vi "main.vi"() -> ()   [LabVIEW 2013]
uses:
  measure/meas session.ctl
  measure/Meas Sweep Config.ctl
  measure/Meas Freq Info.ctl
  measure/meas_swp_mode.ctl
  measure/meas_sweep_flist_mode.ctl
  bridge/Bridge Session.ctl
  bridge/Bridge Type.ctl
  drivers/TWM client/TWM Session.ctl
  drivers/TWM client/TWM parameters.ctl
  drivers/TWM client/Meas Proc QWTB Uncertainty Mode.ctl
  source/Source Session.ctl
  source/Source Type.ctl
  drivers/AFG3101C/AFG3101C Session.ctl
  drivers/cDAQ DDS/cDAQ DDS Session.ctl
  drivers/cDAQ DDS/cDAQ DDS Setup.ctl
  drivers/Fluke 5XXX/top_lev/F5xxx_session.ctl
  drivers/Fluke 5XXX/top_lev/F5xxx_output_mode.ctl
  measure/Meas Results.ctl
  bridge/Bridge Frequency Readings Data.ctl
  drivers/TWM client/Meas Proc QWTB Spectrum Data.ctl
  measure/Meas Result GUI References.ctl
  measure/Meas Result Freq Format.ctl
  measure/Meas Results Sweep Data Uncertainty Mode.ctl
  measure/Meas Result 4TP Impedance Mode.ctl
  measure/Meas Result Major Format.ctl
  measure/Meas Result Deviation Format.ctl
  varilib/SGUI Assign References Mode.ctl
  varilib/SGUI Assign Multiple Strings With Tags By Label.vi
  varilib/varilib.lvlib
panel:
  in  "mode 4TP":T1 caption="4TP display mode"
  in  "unc mode":T2 caption="Uncertainty display mode"
  in  "res frq fmt":T3
  in  "mnr dev fmt":T4 caption="Enum"
  in  "mjr dev fmt":T4 caption="Enum"
  in  "mnr fmt":T5=enum."%_5p"
  in  "mjr fmt":T5=enum."%_5p"
  out "tab swp":string[][](table) caption="Sweep data"
  out "gui refs":T6
  in  "results":T7
  out "meas ref":refnum<vi>
  in  "grp tabs":enum32{"Z", "Z(f)", "FFT", "Info"}(tab)
  out "grp Z mnr":dbl[](graph) caption="minor"
  out "grp Z mjr":dbl[](graph) caption="major"
  in  "swp mnr log":bool caption="Log"
  out "grp swp Z mnr":cluster{dbl[], dbl[]}[](graph) caption="minor"
  out "grp swp Z mjr":cluster{dbl[], dbl[]}[](graph) caption="major"
  in  "swp mjr log":bool caption="Log"
  out "grp ref":string
  out "grp spec 1":cluster{dbl[], dbl[]}(graph) caption="Amplitude spectrum for chn. 1"
  out "grp spec 0":cluster{dbl[], dbl[]}(graph) caption="Amplitude spectrum for chn. 0"
  in  "cb spec log":bool=TRUE caption="Log frequency"
  out "idn src":string caption="Source identifier"
  out "idn brg":string caption="Bridge/digitizers identifier"
  out "open cor":string caption="Open correction file"
  out "short cor":string caption="Short correction file"
  in  "swp com":string caption="Measurement comment"
  out "cab cor":string caption="Cable correction file"
  out "mpx cor":string caption="Multiplexer correction file"
  in  "fgen volts":string[][](table)=[["", "", ""]] caption="F-gen voltages"
  in  "meas":T10={"swp cfg"={"N"=0, "R"=0, "f list"=[], "smpl delay"=0.0, "set delay"=0.0, "set delay np"=0.0, "meas root"=path "", "meas name"="", "meas a-index"=FALSE, "rnd sweep"=FALSE, "mode"=enum."Frequency", "swp mode"=enum."Linear", "avg"=0, "subrec"=0}, "bridge"={"type"=enum."TWM client", "TWM"={"pipe name"="", "parameters"=[], "handle"=0, "fixed aper [s]"=0.0, "f-list [Hz]"=[], "discrete f-list"=FALSE, "unc mode"=enum."None", "unc mcc"=0, "unc first"=FALSE}, "last f"=0.0}, "src"={"type"=enum."Tektronix AFG3101C", "afg"={"VISA"="", "const"=0.0, "gen DC"=FALSE}, "cDAQ dds"={"device"="", "channels"=[], "mclk source"="", "mclk [Hz]"=0.0, "use ext mclk"=FALSE, "fs [Hz]"=0.0, "block [s]"=0.0, "buf [s]"=0.0, "task"="", "cmd queue"=refnum, "proc ref"=refnum, "smpl clock out"="/cDAQ3/PFI0", "export smpl clock"=FALSE}, "gain [V/A]"=1.0, "F5xxx session"={"VISA"="", "mode"=enum."AC voltage", "Earth on"=FALSE, "Ext ref lock"=FALSE}}, "results"=refnum} {"src"."cDAQ dds"."channels" min=0 step=1; "bridge"."TWM"."f-list [Hz]" format="%#_6p"; "swp cfg"."f list"."bias" format="%#_3p"; "swp cfg"."f list"."level" format="%#_3p"; "swp cfg"."f list"."fs [Hz]" format="%#_5p"; "swp cfg"."f list"."time [s]" format="%#_3p"; "swp cfg"."f list"."f/fs" format="%#_3p"; "swp cfg"."f list"."periods" format="%#_3f"; "swp cfg"."f list"."f [Hz]" format="%#_5p"}
  out "error":errorcluster
  in  "btn exit":bool
  in  "btn set&start":bool
  in  "btn cfg src":bool
  in  "btn cfg adc":bool
  in  "btn stop":bool
  out "stat3":string
  out "stat2":string
  out "stat1":string
  in  "btn about":bool
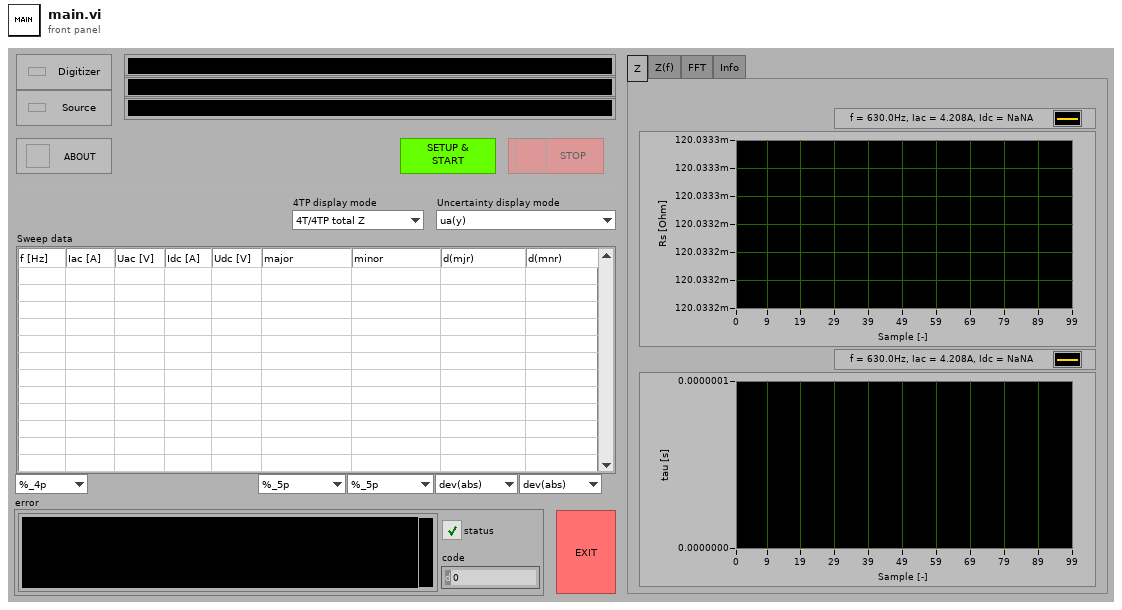
[diagram p1: front panel]
types:
  T1 = typedef "Meas Result 4TP Impedance Mode.ctl" = enum16{"4T/4TP total Z", "4TP-shield Z"}
  T2 = typedef "Meas Results Sweep Data Uncertainty Mode.ctl" = enum16{"ua(y)", "ua(y) (p=95%)", "uc(y) (p=95%)"}
  T3 = typedef "Meas Result Freq Format.ctl" = enum16{"%_4p", "%_4f"}
  T4 = typedef "Meas Result Deviation Format.ctl" = enum16{"dev(abs)", "dev(%)", "dev(ppm)", "u(abs)", "u(%)", "u(ppm)"}
  T5 = typedef "Meas Result Major Format.ctl" = enum16{"%_3p", "%_4p", "%_5p", "%_6p", "%_7p", "%_8p", "%_5f", "%_6f", "%_7f", "%_8f"}
  T6 = typedef "Meas Result GUI References.ctl" = cluster{"grp Z mjr":refnum<vi>, "grp Z mnr":refnum<vi>, "grp swp Z mjr":refnum<vi>, "grp swp Z mnr":refnum<vi>, "swp mjr log":refnum<vi>, "swp mnr log":refnum<vi>, "grp ref":refnum<vi>, "tab swp":refnum<vi>, "mjr fmt":refnum<vi>, "mnr fmt":refnum<vi>, "mjr dev fmt":refnum<vi>, "mnr dev fmt":refnum<vi>, "res frq fmt":refnum<vi>, "unc mode":refnum<vi>, "mode 4TP":refnum<vi>, "grp spec 0":refnum<vi>, "grp spec 1":refnum<vi>, "cb spec log":refnum<vi>}
  T7 = typedef "Meas Results.ctl" = cluster{"freqs":T8[], "locked":bool, "last fid":i32, "modified":bool, "mjr name":string, "mnr name":string, "last spectra":T9[]}
  T8 = typedef "Bridge Frequency Readings Data.ctl" = cluster{"Udut":dbl[], "Iref":dbl[], "Udc":dbl[], "Idc":dbl[], "mjr":dbl[], "mnr":dbl[], "mjr_sh":dbl[], "mnr_sh":dbl[], "u(mjr)":dbl[], "u(mnr)":dbl[], "ua2(mjr)":dbl[], "ua2(mnr)":dbl[], "n":i32, "f [Hz]":dbl}
  T9 = typedef "Meas Proc QWTB Spectrum Data.ctl" = cluster{"x":sgl[], "y":sgl[], "label":string}
  T10 = typedef "meas session.ctl" = cluster{"swp cfg":T11, "bridge":T15, "src":T20, "results":refnum<vi>}
  T11 = typedef "Meas Sweep Config.ctl" = cluster{"N":i32, "R":i32, "f list":T12[], "smpl delay":dbl, "set delay":dbl, "set delay np":dbl, "meas root":path, "meas name":string, "meas a-index":bool, "rnd sweep":bool, "mode":T13, "swp mode":T14, "avg":i32, "subrec":i32}
  T12 = typedef "Meas Freq Info.ctl" = cluster{"f [Hz]":dbl, "periods":dbl, "f/fs":dbl, "time [s]":dbl, "fs [Hz]":dbl, "N":i32, "level":dbl, "bias":dbl}
  T13 = typedef "meas_swp_mode.ctl" = enum16{"Frequency", "Level", "Bias"}
  T14 = typedef "meas_sweep_flist_mode.ctl" = enum16{"Linear", "Log10"}
  T15 = typedef "Bridge Session.ctl" = cluster{"type":T16, "TWM":T17, "last f":dbl}
  T16 = typedef "Bridge Type.ctl" = enum16{"TWM client", "dummy"}
  T17 = typedef "TWM Session.ctl" = cluster{"pipe name":string, "parameters":T18[], "handle":i32, "fixed aper [s]":dbl, "f-list [Hz]":dbl[], "discrete f-list":bool, "unc mode":T19, "unc mcc":i32, "unc first":bool}
  T18 = typedef "TWM parameters.ctl" = cluster{"name":string, "value":string[]}
  T19 = typedef "Meas Proc QWTB Uncertainty Mode.ctl" = enum16{"None", "GUF", "Monte Carlo"}
  T20 = typedef "Source Session.ctl" = cluster{"type":T21, "afg":T22, "cDAQ dds":T23, "gain [V/A]":dbl, "F5xxx session":T24}
  T21 = typedef "Source Type.ctl" = enum16{"Tektronix AFG3101C", "cDAQ DAC", "Fluke 5xxx", "dummy"}
  T22 = typedef "AFG3101C Session.ctl" = cluster{"VISA":refnum<visa-resource-name>, "const":dbl, "gen DC":bool}
  T23 = typedef "cDAQ DDS Session.ctl" = cluster{"device":tag, "channels":i32[], "mclk source":tag, "mclk [Hz]":dbl, "use ext mclk":bool, "fs [Hz]":dbl, "block [s]":dbl, "buf [s]":dbl, "task":refnum<k21>, "cmd queue":refnum<queue>, "proc ref":refnum<vi>, "smpl clock out":tag, "export smpl clock":bool}
  T24 = typedef "F5xxx_session.ctl" = cluster{"VISA":refnum<visa-resource-name>, "mode":T25, "Earth on":bool, "Ext ref lock":bool}
  T25 = typedef "F5xxx_output_mode.ctl" = enum16{"AC voltage", "AC current"}
  T26 = typedef "varilib.lvlib/SGUI Assign References Mode.ctl" = enum16{"Add to stack", "Overwrite", "Release last", "Release ID"}
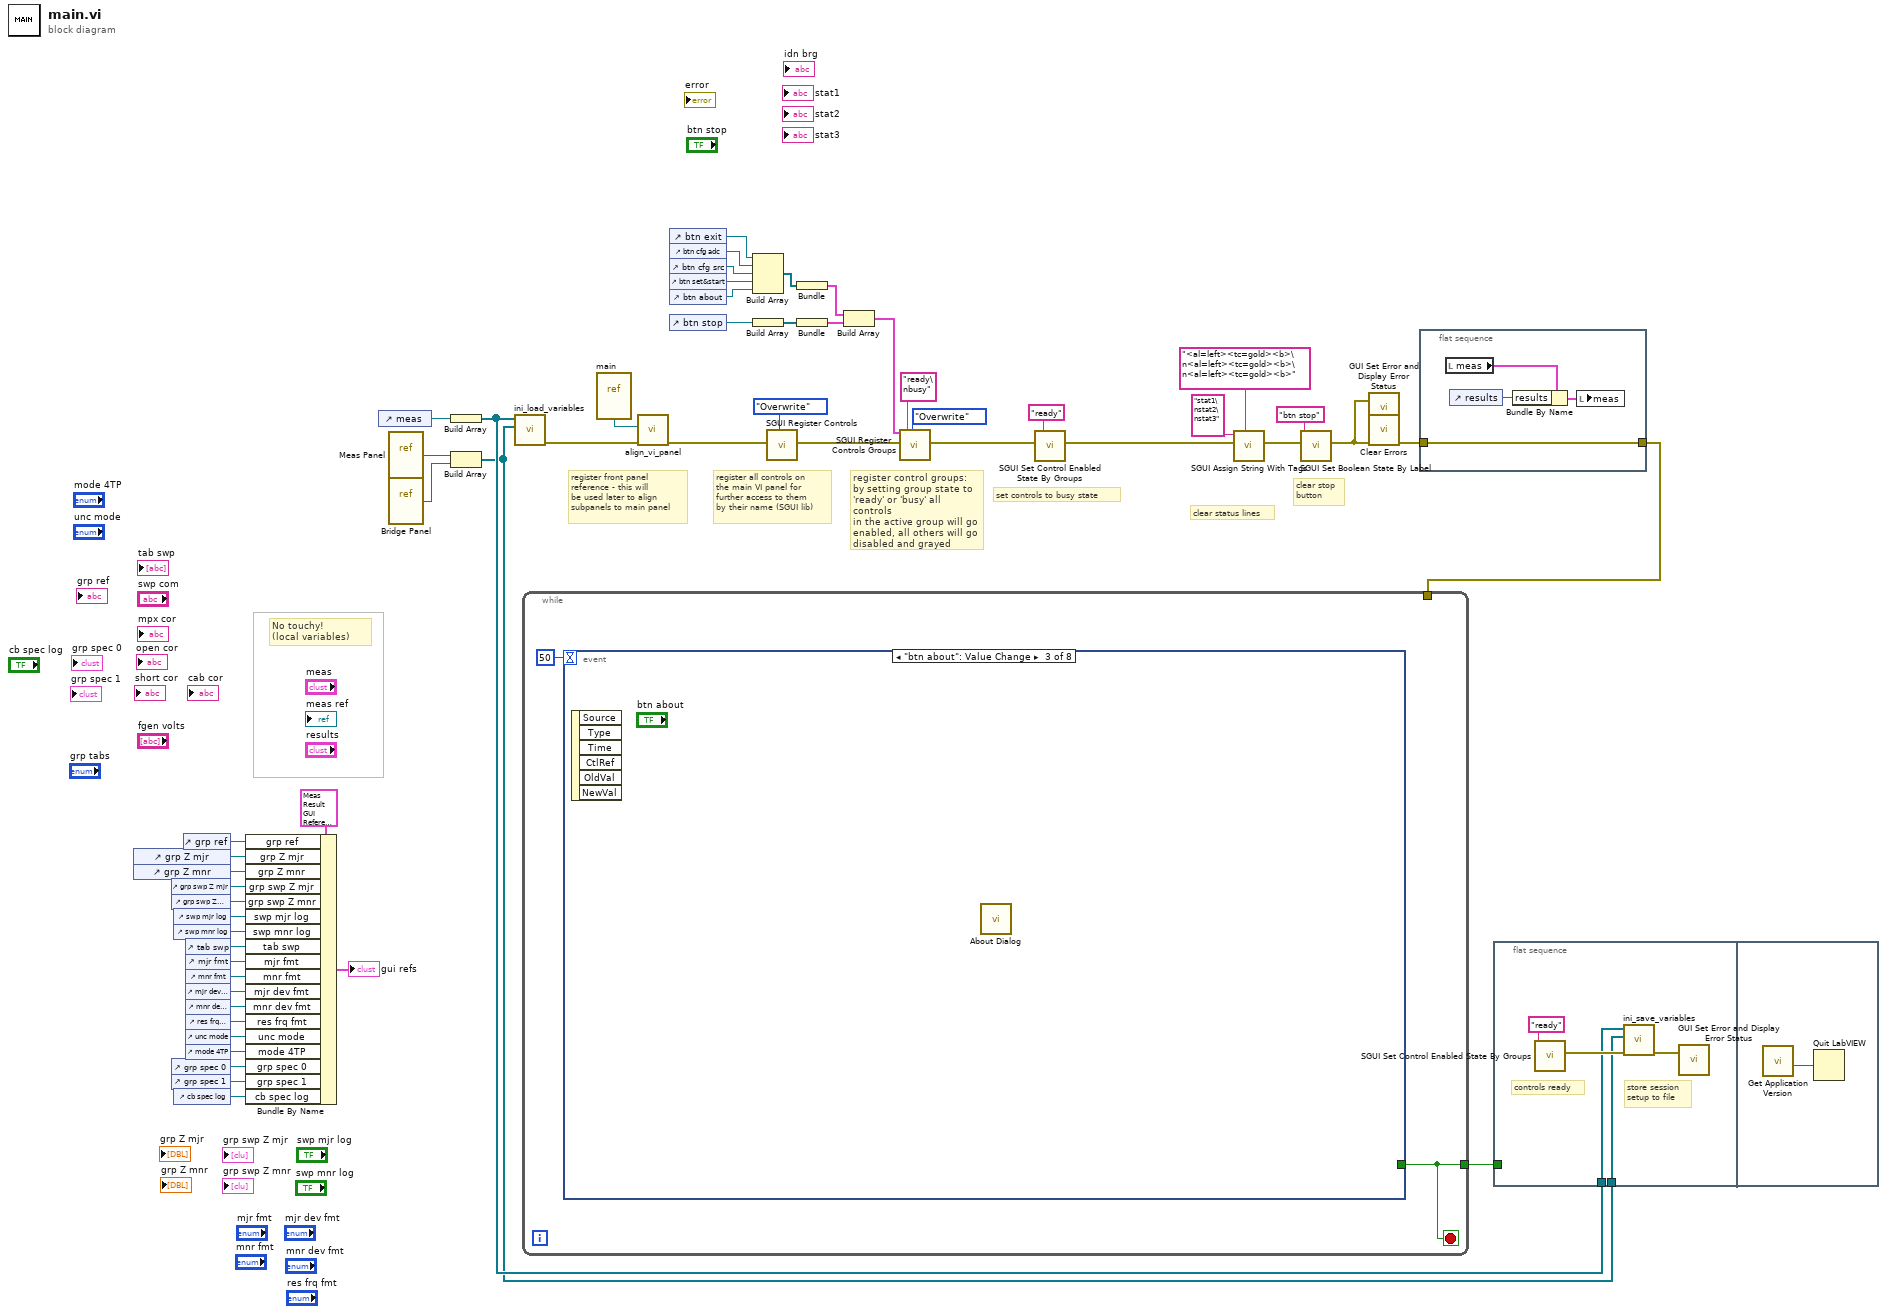
[diagram p0: block diagram]
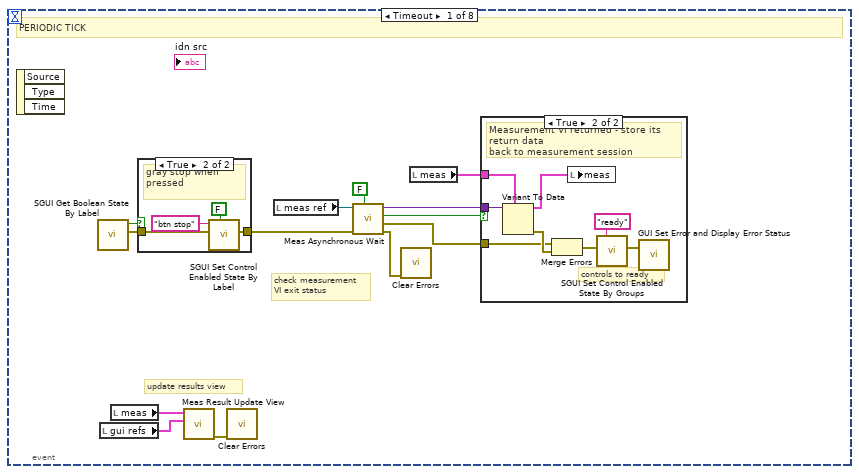
[diagram p2: hidden frame]
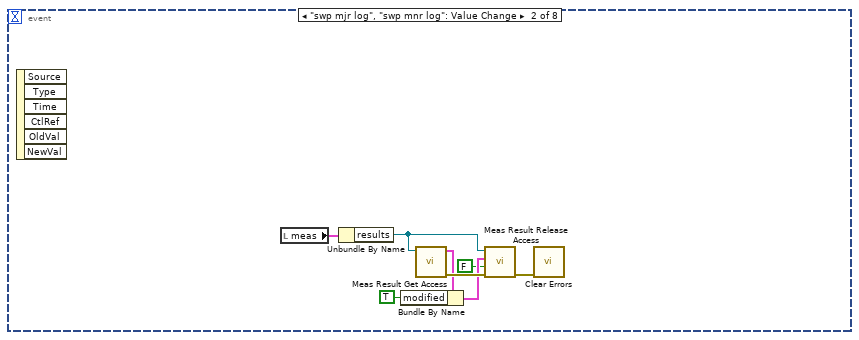
[diagram p5: hidden frame]
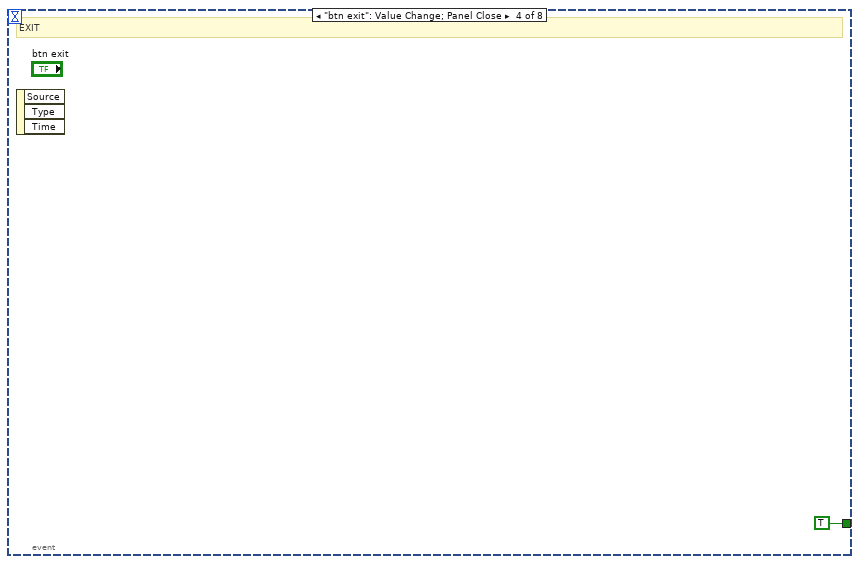
[diagram p6: hidden frame]
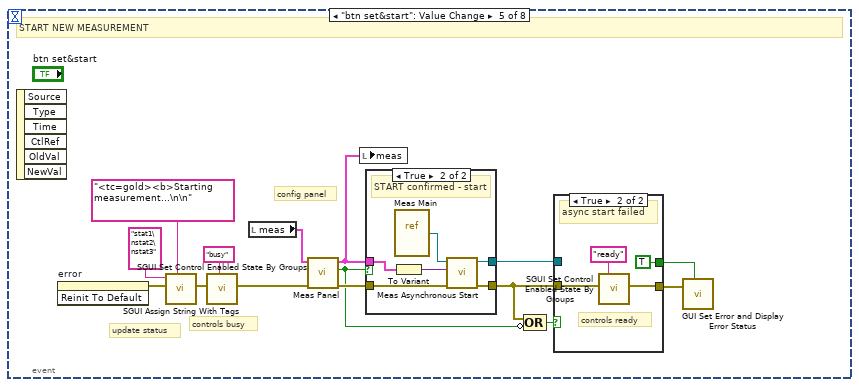
[diagram p7: hidden frame]
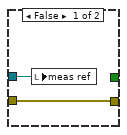
[diagram p8: hidden frame]
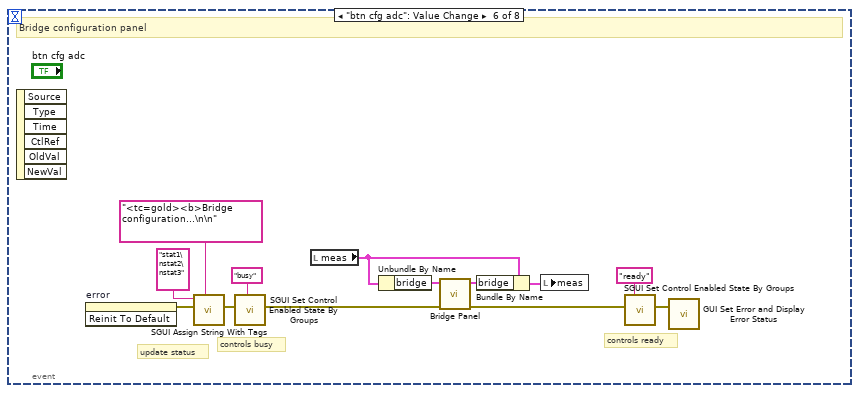
[diagram p10: hidden frame]
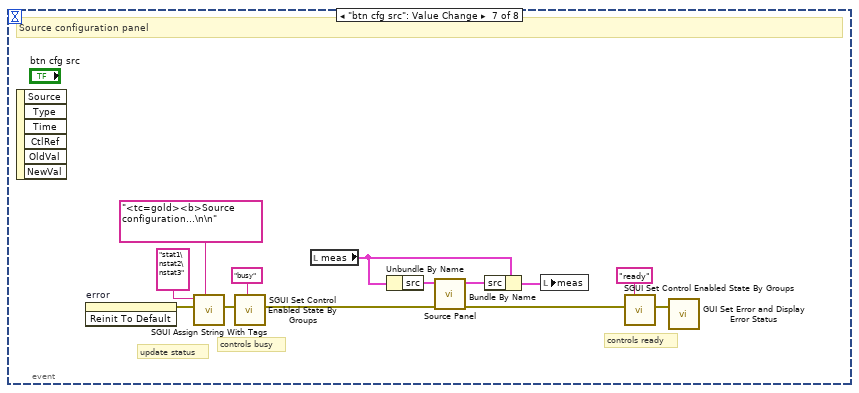
[diagram p11: hidden frame]
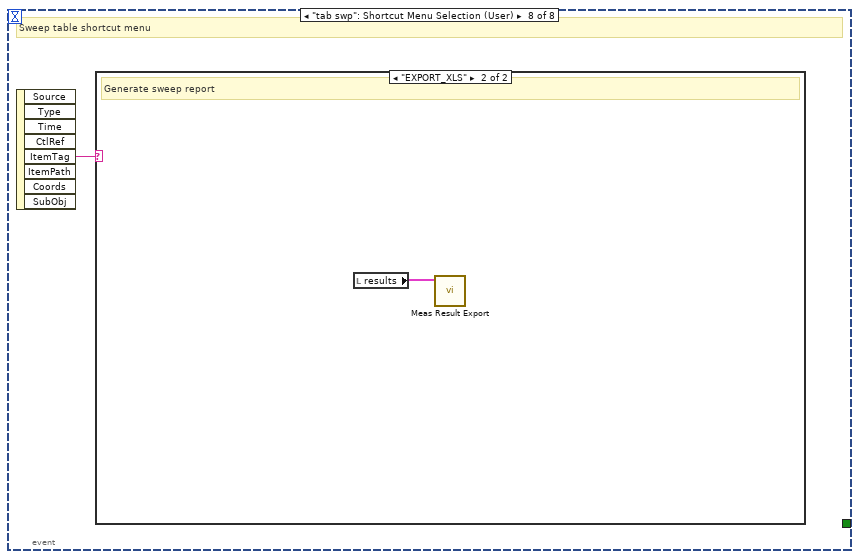
[diagram p12: hidden frame]
diagram:
  # "No touchy!\n(local variables)"
  # "clear status lines"
  # "register front panel\nreference - this will\nbe used later to align\nsubpanels to main panel"
  # "clear stop\nbutton"
  # "set controls to busy state"
  # "register control groups:\nby setting group state to\n'ready' or 'busy' all controls\nin the active group will go\nenabled, all others will go\ndisabled and grayed"
  # "register all controls on\nthe main VI panel for \nfurther access to them\nby their name (SGUI lib)"
  n1 = control-ref of="grp Z mjr"() -> (w19:refnum<vi>)
  n2 = control-ref of="grp Z mnr"() -> (w18:refnum<vi>)
  n3 = control-ref of="grp swp Z mjr"() -> (w17:refnum<vi>)
  n4 = control-ref of="grp swp Z mnr"() -> (w16:refnum<vi>)
  n5 = control-ref of="grp spec 0"() -> (w3:refnum<vi>)
  n6 = control-ref of="grp spec 1"() -> (w2:refnum<vi>)
  n7 = control-ref of="swp mjr log"() -> (w15:refnum<vi>)
  n8 = control-ref of="swp mnr log"() -> (w14:refnum<vi>)
  n9 = control-ref of="cb spec log"() -> (w1:refnum<vi>)
  n10 = control-ref of="grp ref"() -> (w12:refnum<vi>)
  n11 = control-ref of="tab swp"() -> (w11:refnum<vi>)
  n12 = control-ref of="mjr fmt"() -> (w10:refnum<vi>)
  n13 = control-ref of="mnr fmt"() -> (w9:refnum<vi>)
  n14 = control-ref of="mjr dev fmt"() -> (w8:refnum<vi>)
  n15 = control-ref of="mnr dev fmt"() -> (w7:refnum<vi>)
  n16 = control-ref of="res frq fmt"() -> (w6:refnum<vi>)
  n17 = control-ref of="unc mode"() -> (w5:refnum<vi>)
  n18 = control-ref of="mode 4TP"() -> (w4:refnum<vi>)
  n19 = Bundle By Name(cluster=T6 {"grp Z mjr"=refnum, "grp Z mnr"=refnum, "grp swp Z mjr"=refnum, "grp swp Z mnr"=refnum, "swp mjr log"=refnum, "swp mnr log"=refnum, "grp ref"=refnum, "tab swp"=refnum, "mjr fmt"=refnum, "mnr fmt"=refnum, "mjr dev fmt"=refnum, "mnr dev fmt"=refnum, "res frq fmt"=refnum, "unc mode"=refnum, "mode 4TP"=refnum, "grp spec 0"=refnum, "grp spec 1"=refnum, "cb spec log"=refnum} ("res gui ref"), "grp ref"=w12, "grp Z mjr"=w19, "grp Z mnr"=w18, "grp swp Z mjr"=w17, "grp swp Z mnr"=w16, "swp mjr log"=w15, "swp mnr log"=w14, "tab swp"=w11, "mjr fmt"=w10, "mnr fmt"=w9, "mjr dev fmt"=w8, "mnr dev fmt"=w7, "res frq fmt"=w6, "unc mode"=w5, "mode 4TP"=w4, "grp spec 0"=w3, "grp spec 1"=w2, "cb spec log"=w1) -> (→"gui refs":T6)
  n20 = control-ref of="meas"() -> (w41:refnum<vi>)
  n21 = vi-ref "Meas Panel.vi"() -> (w27:refnum<vi>)
  n22 = vi-ref "Bridge Panel.vi"() -> (w25:refnum<vi>)
  n23 = Build Array(w41) -> (w40:refnum<vi>[])
  n24 = Build Array(w27, w25) -> (w26:refnum<vi>[])
  n25 = call "ini_load_variables.vi"("VI to store"=w26, "objects to store"=w40) -> ("error out"=w42:errorcluster)  [unwired: 9 in]
  n26 = while {
    tunnel: w21 -> [_]
    tunnel: [w56] -> w28
    stop <- w56 stop-if-true
    n27 = event shown="[2] \"btn about\": Value Change" {
      selector: _ -> [_ _ _ _ _ _ _ _]
      dyn-events: _ -> [_ _ _ _ _ _ _ _]
      timeout: 50 -> [_ _ _ _ _ _ _ _]
      tunnel: [_ _ _ TRUE _ _ _ _] -> w56
      event Timeout {
        # "update results view"
        # "check measurement\nVI exit status"
        # "PERIODIC TICK"
        n28 = event-data() -> ()  [unwired: 1 in, 3 out]
        n29 = call "SGUI Get Boolean State By Label.vi"() -> ("error out"=w69:errorcluster, "binary state out"=w68:bool)  [unwired: 9 in, 1 out]
        n30 = local read "gui refs"() -> (w58:T6)
        n31 = local read "meas"() -> (w59:T10)
        n32 = case shown="True" w68 {
          tunnel: w69 -> [w78 w82]
          tunnel: [w78 w80] -> w64
          frame False {
          }
          frame True {
            # "gray stop when\npressed"
            n33 = call "SGUI Set Control Enabled State By Label.vi"("error in"=w82, "labels (empty)"="btn stop", "Enabled? (False)"=FALSE) -> ("error out"=w80:errorcluster)  [unwired: 7 in, 1 out]
          }
        }
        n34 = call "Meas Result Update View.vi"("gui refs"=w58, "meas"=w59) -> ("error out"=w57:errorcluster)  [unwired: 9 in]
        n35 = call <vilib>:"Clear Errors.vi"("error in (no error)"=w57) -> ()  [unwired: 6 in, 1 out]
        n36 = local read "meas ref"() -> (w65:refnum<vi>)
        n37 = call "Meas Asynchronous Wait.vi"("Wait for exit? (False)"=FALSE, "error in"=w64, "VI reference (empty)"=w65) -> ("error out"=w67:errorcluster, "VI's error out"=w61:errorcluster, "VI returned?"=w62:bool, "parameter out"=w63:variant)  [unwired: 4 in, 1 out]
        n38 = call <vilib>:"Clear Errors.vi"("error in (no error)"=w67) -> ()  [unwired: 6 in, 1 out]
        n39 = local read "meas"() -> (w60:T10)
        n40 = case shown="True" w62 {
          tunnel: w63 -> [_ w70]
          tunnel: w61 -> [_ w74]
          tunnel: w60 -> [_ w73]
          frame False {
          }
          frame True {
            # "controls to ready"
            # "Measurement VI returned - store its return data\nback to measurement session"
            n41 = Variant To Data(type=w73, Variant=w70) -> (data=w71:T10, error out=w77:errorcluster)  [unwired: 1 in]
            n42 = Merge Errors(w74, w77) -> (w76:errorcluster)
            n43 = local write "meas"(w71) -> ()
            n44 = call "SGUI Set Control Enabled State By Groups.vi"("error in"=w76, "group name to enable (none)"="ready") -> ("error out"=w72:errorcluster)  [unwired: 8 in, 1 out]
            n45 = call "GUI Set Error and Display Error Status.vi"("error in"=w72) -> ()  [unwired: 4 in]
          }
        }
      }
      event "swp mjr log", "swp mnr log": Value Change {
        n46 = event-data() -> ()  [unwired: 1 in, 6 out]
        n47 = local read "meas"() -> (w84:T10)
        n48 = Unbundle By Name(w84) -> ("results"=w89:refnum<vi>)
        n49 = call "Meas Result Get Access.vi"("results ref"=w89) -> ("error out"=w90:errorcluster, "results data"=w86:T7)  [unwired: 9 in]
        n50 = Bundle By Name(cluster=w86, "modified"=TRUE) -> (w88:T7)
        n51 = call "Meas Result Release Access.vi"("error in"=w90, "Release only (True)"=FALSE, "results data in"=w88, "results ref"=w89) -> ("error out"=w85:errorcluster)  [unwired: 7 in]
        n52 = call <vilib>:"Clear Errors.vi"("error in (no error)"=w85) -> ()  [unwired: 6 in, 1 out]
      }
      event "btn about": Value Change {
        n53 = event-data() -> ()  [unwired: 1 in, 6 out]
        n54 = call "About Dialog.vi"() -> ()  [unwired: 12 in]
      }
      event "btn exit": Value Change; Panel Close {
        # "EXIT"
        n55 = event-data() -> ()  [unwired: 1 in, 3 out]
      }
      event "btn set&start": Value Change {
        # "config panel"
        # "update status"
        # "controls busy"
        # "START NEW MEASUREMENT"
        n56 = event-data() -> ()  [unwired: 1 in, 6 out]
        n57 = invoke on="error" class="Clust (strict)" method="Reinit To Default"() -> (error out=w102:errorcluster)  [unwired: 3 in, 2 out]
        n58 = call-poly "SGUI Assign String With Tags.vi"("error in"=w102, "label(s) (empty)"="stat1\nstat2\nstat3", "string (empty)"="<tc=gold><b>Starting measurement...\n\n") -> ("error out"=w104:errorcluster)  [unwired: 7 in, 1 out]
        n59 = call "SGUI Set Control Enabled State By Groups.vi"("error in"=w104, "group name to enable (none)"="busy") -> ("error out"=w101:errorcluster)  [unwired: 8 in, 1 out]
        n60 = local read "meas"() -> (w99:T10)
        n61 = call "Meas Panel.vi"("error in"=w101, "meas in"=w99) -> ("error out"=w100:errorcluster, "OK"=w95:bool, "meas out"=w98:T10)  [unwired: 7 in]
        n62 = local write "meas"(w98) -> ()
        n63 = case shown="True" w95 {
          tunnel: w100 -> [w113 w119]
          tunnel: w98 -> [_ w117]
          tunnel: [w113 w116] -> w96
          tunnel: [_ w114] -> w94
          frame False {
          }
          frame True {
            # "START confirmed - start"
            n64 = To Variant(anything=w117) -> (Variant=w118:variant)
            n65 = vi-ref "Meas Main.vi"() -> (w115:refnum<vi>)
            n66 = call "Meas Asynchronous Start.vi"("error in"=w119, "parameter in"=w118, "Static VI reference in (empty)"=w115) -> ("error out"=w116:errorcluster, "async VI reference out"=w114:refnum<vi>)  [unwired: 7 in]
          }
        }
        n67 = Compound Arithmetic op=OR(w96, invert w95) -> (w97:bool)
        n68 = case shown="True" w97 {
          tunnel: w96 -> [w107 w111]
          tunnel: [w107 w110] -> w93
          tunnel: w94 -> [w108 _]
          tunnel: [_ TRUE] -> w92
          frame False {
            n69 = local write "meas ref"(w108) -> ()
          }
          frame True {
            # "controls ready"
            # "async start failed"
            n70 = call "SGUI Set Control Enabled State By Groups.vi"("error in"=w111, "group name to enable (none)"="ready") -> ("error out"=w110:errorcluster)  [unwired: 8 in, 1 out]
          }
        }
        n71 = call "GUI Set Error and Display Error Status.vi"("error in"=w93, "Write status only if error occures? (False)"=w92) -> ()  [unwired: 3 in]
      }
      event "btn cfg adc": Value Change {
        # "controls ready"
        # "update status"
        # "controls busy"
        # "Bridge configuration panel"
        n72 = event-data() -> ()  [unwired: 1 in, 6 out]
        n73 = invoke on="error" class="Clust (strict)" method="Reinit To Default"() -> (error out=w128:errorcluster)  [unwired: 3 in, 2 out]
        n74 = call-poly "SGUI Assign String With Tags.vi"("error in"=w128, "label(s) (empty)"="stat1\nstat2\nstat3", "string (empty)"="<tc=gold><b>Bridge configuration...\n\n") -> ("error out"=w130:errorcluster)  [unwired: 7 in, 1 out]
        n75 = call "SGUI Set Control Enabled State By Groups.vi"("error in"=w130, "group name to enable (none)"="busy") -> ("error out"=w125:errorcluster)  [unwired: 8 in, 1 out]
        n76 = local read "meas"() -> (w122:T10)
        n77 = Unbundle By Name(w122) -> ("bridge"=w123:T15)
        n78 = call "Bridge Panel.vi"("error in"=w125, "bridge in"=w123) -> ("error out"=w124:errorcluster, "bridge out"=w121:T15)  [unwired: 8 in]
        n79 = Bundle By Name(cluster=w122, "bridge"=w121) -> (w120:T10)
        n80 = local write "meas"(w120) -> ()
        n81 = call "SGUI Set Control Enabled State By Groups.vi"("error in"=w124, "group name to enable (none)"="ready") -> ("error out"=w127:errorcluster)  [unwired: 8 in, 1 out]
        n82 = call "GUI Set Error and Display Error Status.vi"("error in"=w127) -> ()  [unwired: 4 in]
      }
      event "btn cfg src": Value Change {
        # "controls ready"
        # "update status"
        # "controls busy"
        # "Source configuration panel"
        n83 = event-data() -> ()  [unwired: 1 in, 6 out]
        n84 = invoke on="error" class="Clust (strict)" method="Reinit To Default"() -> (error out=w141:errorcluster)  [unwired: 3 in, 2 out]
        n85 = call-poly "SGUI Assign String With Tags.vi"("error in"=w141, "label(s) (empty)"="stat1\nstat2\nstat3", "string (empty)"="<tc=gold><b>Source configuration...\n\n") -> ("error out"=w143:errorcluster)  [unwired: 7 in, 1 out]
        n86 = call "SGUI Set Control Enabled State By Groups.vi"("error in"=w143, "group name to enable (none)"="busy") -> ("error out"=w136:errorcluster)  [unwired: 8 in, 1 out]
        n87 = local read "meas"() -> (w138:T10)
        n88 = Unbundle By Name(w138) -> ("src"=w135:T20)
        n89 = call "Source Panel.vi"("error in"=w136, "src in"=w135) -> ("error out"=w133:errorcluster, "src out"=w134:T20)  [unwired: 8 in]
        n90 = Bundle By Name(cluster=w138, "src"=w134) -> (w137:T10)
        n91 = local write "meas"(w137) -> ()
        n92 = call "SGUI Set Control Enabled State By Groups.vi"("error in"=w133, "group name to enable (none)"="ready") -> ("error out"=w140:errorcluster)  [unwired: 8 in, 1 out]
        n93 = call "GUI Set Error and Display Error Status.vi"("error in"=w140) -> ()  [unwired: 4 in]
      }
      event "tab swp": Shortcut Menu Selection (User) {
        # "Sweep table shortcut menu"
        n94 = event-data() -> ("ItemTag"=w146:string)  [unwired: 1 in, 7 out]
        n95 = case shown="\"EXPORT_XLS\"" w146 {
          frame Default {
          }
          frame "EXPORT_XLS" {
            # "Generate sweep report"
            n96 = local read "results"() -> (w147:T7)
            n97 = call "Meas Result Export.vi"("result"=w147) -> ()  [unwired: 10 in, 1 out]
          }
        }
      }
    }
  }
  n98 = vi-ref "main.vi"() -> (w43:refnum<vi>)
  n99 = call "align_vi_panel.vi"("error in"=w42, "top vi reference"=w43) -> ("error out"=w47:errorcluster)  [unwired: 9 in]
  n100 = control-ref of="btn exit"() -> (w29:refnum<vi>)
  n101 = control-ref of="btn cfg adc"() -> (w30:refnum<vi>)
  n102 = control-ref of="btn cfg src"() -> (w31:refnum<vi>)
  n103 = control-ref of="btn set&start"() -> (w35:refnum<vi>)
  n104 = control-ref of="btn about"() -> (w34:refnum<vi>)
  n105 = control-ref of="btn stop"() -> (w37:refnum<vi>)
  n106 = Build Array(w29, w30, w31, w35, w34) -> (w33:refnum<vi>[])
  n107 = Build Array(w37) -> (w32:refnum<vi>[])
  n108 = call "SGUI Register Controls.vi"("error in"=w47, "register mode (overwrite)"=SGUI_Assign_References_Mode."Overwrite") -> ("error out"=w53:errorcluster)  [unwired: 15 in, 2 out]
  n109 = Bundle(w33) -> (w38:cluster{refnum<vi>[]})  [unwired: 1 in]
  n110 = Bundle(w32) -> (w36:cluster{refnum<vi>[]})  [unwired: 1 in]
  n111 = Build Array(w38, w36) -> (w39:cluster{refnum<vi>[]}[])
  n112 = call "SGUI Register Controls Groups.vi"("control groups"=w39, "error in"=w53, "groups names"="ready\nbusy", "register mode (overwrite)"=SGUI_Assign_References_Mode."Overwrite") -> ("error out"=w50:errorcluster)  [unwired: 14 in, 1 out]
  n113 = call "SGUI Set Control Enabled State By Groups.vi"("error in"=w50, "group name to enable (none)"="ready") -> ("error out"=w23:errorcluster)  [unwired: 8 in, 1 out]
  n114 = call-poly "SGUI Assign String With Tags.vi"("error in"=w23, "label(s) (empty)"="stat1\nstat2\nstat3", "string (empty)"="<al=left><tc=gold><b>\n<al=left><tc=gold><b>\n<al=left><tc=gold><b>") -> ("error out"=w44:errorcluster)  [unwired: 7 in, 1 out]
  n115 = call "SGUI Set Boolean State By Label.vi"("error in"=w44, "control label(s) ('btn stop')"="btn stop") -> ("error out"=w24:errorcluster)  [unwired: 8 in, 1 out]
  n116 = call "GUI Set Error and Display Error Status.vi"("error in"=w24) -> ()  [unwired: 4 in]
  n117 = call <vilib>:"Clear Errors.vi"("error in (no error)"=w24) -> ("error out"=w22:errorcluster)  [unwired: 6 in]
  n118 = flat-sequence {
    tunnel: w22 -> [w151]
    tunnel: [w151] -> w21
    frame #0 {
      n119 = local read "meas"() -> (w148:T10)
      n120 = control-ref of="results"() -> (w150:refnum<vi>)
      n121 = Bundle By Name(cluster=w148, "results"=w150) -> (w149:T10)
      n122 = local write "meas"(w149) -> ()
    }
  }
  n123 = flat-sequence {
    tunnel: w40 -> [w154]
    tunnel: w28 -> [_]
    tunnel: w26 -> [w153]
    frame #0 {
      # "store session\nsetup to file"
      # "controls ready"
      n124 = call "SGUI Set Control Enabled State By Groups.vi"("group name to enable (none)"="ready") -> ("error out"=w155:errorcluster)  [unwired: 9 in, 1 out]
      n125 = call "ini_save_variables.vi"("error in"=w155, "VI to store"=w153, "objects"=w154) -> ("error out"=w152:errorcluster)  [unwired: 8 in]
      n126 = call "GUI Set Error and Display Error Status.vi"("error in"=w152) -> ()  [unwired: 4 in]
    }
    frame #1 {
      n127 = call "Get Application Version.vi"() -> ("run time system"=w157:bool)  [unwired: 8 in, 3 out]
      n128 = Quit LabVIEW(quit? (T)=w157) -> ()
    }
  }
